vi "Read Joystick.vi"(8 "Joystick Deadbanded Value (default of 0.1)":dbl, 11 "Joystick L 1 DevRef":T1) -> (1 "Joystick L 2 X Axis":dbl, 2 "Joystick L 1 Y Axis":dbl, 3 "Joystick L 1 X Axis":dbl)   [LabVIEW 2014]
uses:
  <vilib>/Rock Robotics/WPI/Joystick/WPI_JoystickDevRef.ctl
  <vilib>/Rock Robotics/WPI/Joystick/WPI_JoystickDeviceEnum.ctl
  Global Variables.vi
  <vilib>/Rock Robotics/WPI/Joystick/WPI_JoystickGetSetRefNum.vi
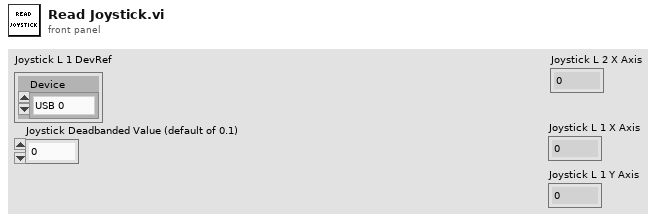
[diagram p1: front panel]
types:
  T1 = typedef "WPI_JoystickDevRef.ctl" = cluster{"Device":T2}
  T2 = typedef "WPI_JoystickDeviceEnum.ctl" = enum16{"USB 0", "USB 1", "USB 2", "USB 3", "USB 4", "USB 5"}
  T3 = cluster{"Buttons[0]":bool, "Buttons[1]":bool, "Buttons[2]":bool, "Buttons[3]":bool, "Buttons[4]":bool, "Buttons[5]":bool, "Buttons[6]":bool, "Buttons[7]":bool, "Buttons[8]":bool}
  T4 = cluster{"Axes[0]":dbl, "Axes[1]":dbl, "Axes[2]":dbl, "Axes[3]":dbl, "Axes[4]":dbl, "Axes[5]":dbl, "Axes[6]":dbl, "Axes[7]":dbl, "Axes[8]":dbl}
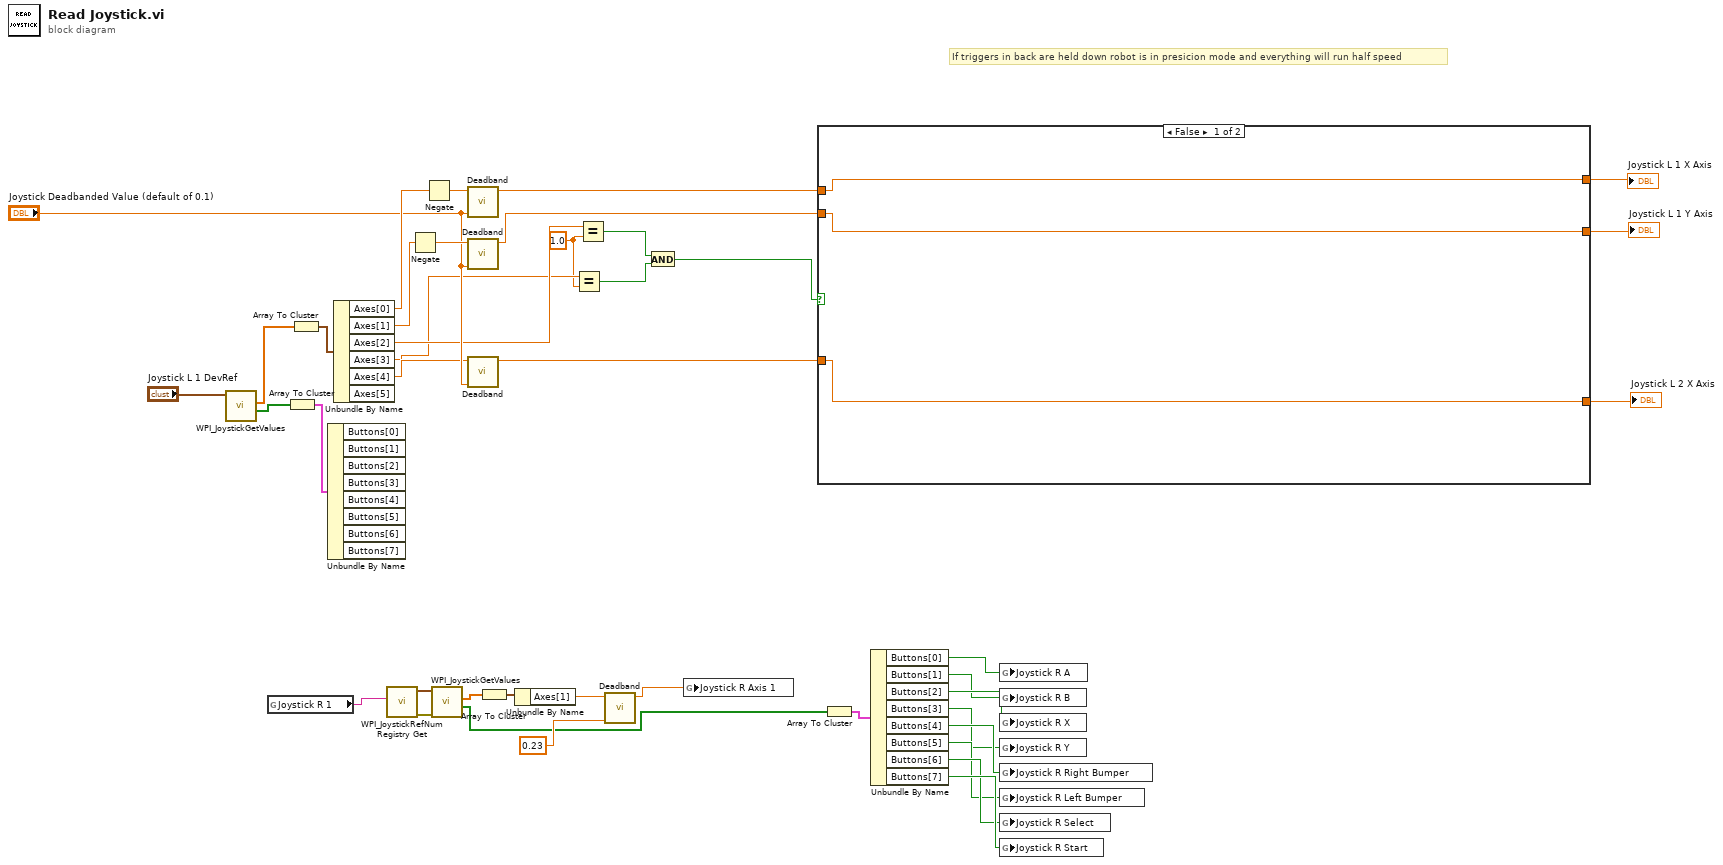
[diagram p0: block diagram]
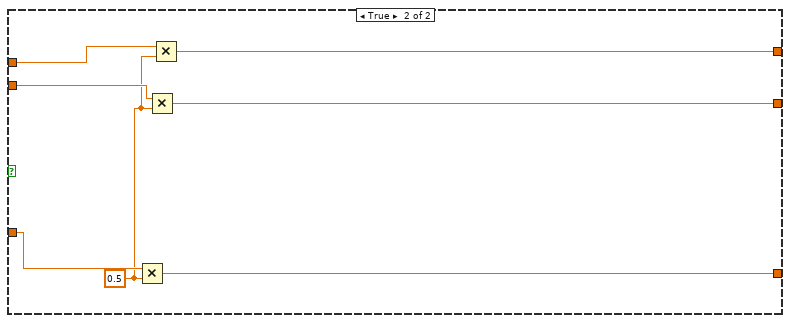
[diagram p2: hidden frame]
diagram:
  w10 = 1.0 ("y")
  # "If triggers in back are held down robot is in presicion mode and everything will run half speed"
  n1 = call <vilib>:"WPI_JoystickGetValues.vi"("JoystickDevRef"="Joystick L 1 DevRef") -> ("Buttons"=w38:bool[], "Axes"=w40:dbl[])  [unwired: 6 in, 3 out]
  n2 = global read "Global Variables.vi" "Joystick R 1"() -> (w29:string)
  n3 = Array To Cluster(array=w38) -> (cluster=w37:T3)
  n4 = Array To Cluster(array=w40) -> (cluster=w39:T4)
  n5 = Unbundle By Name(w37) -> ()  [unwired: 8 out]
  n6 = Unbundle By Name(w39) -> ("Axes[0]"=w36:dbl, "Axes[1]"=w33:dbl, "Axes[2]"=w12:dbl, "Axes[3]"=w11:dbl, "Axes[4]"=w13:dbl)  [unwired: 1 out]
  n7 = call <vilib>:"WPI_JoystickRefNum Registry Get.vi"("refnum name"=w29) -> ("error out"=w28:errorcluster, "JoystickDevRef"=w27:T1)  [unwired: 9 in]
  n8 = Negate(x=w33) -> (-x=w34:dbl)
  n9 = Negate(x=w36) -> (-x=w35:dbl)
  n10 = call <vilib>:"WPI_JoystickGetValues.vi"("error in (no error)"=w28, "JoystickDevRef"=w27) -> ("Buttons"=w15:bool[], "Axes"=w30:dbl[])  [unwired: 5 in, 3 out]
  n11 = call "Deadband.vi"("Value to Deadband (default of 0.1)"="Joystick Deadbanded Value (default of 0.1)", "Value"=w35) -> ("Deadbanded Value"=w4:dbl)  [unwired: 9 in]
  n12 = call "Deadband.vi"("Value to Deadband (default of 0.1)"="Joystick Deadbanded Value (default of 0.1)", "Value"=w34) -> ("Deadbanded Value"=w5:dbl)  [unwired: 9 in]
  n13 = call "Deadband.vi"("Value to Deadband (default of 0.1)"="Joystick Deadbanded Value (default of 0.1)", "Value"=w13) -> ("Deadbanded Value"=w6:dbl)  [unwired: 9 in]
  n14 = Array To Cluster(array=w30) -> (cluster=w31:T4)
  n15 = Unbundle By Name(w31) -> ("Axes[1]"=w25:dbl)
  n16 = Equal?(x=w11, y=w10) -> (x = y?=w8:bool)
  n17 = Equal?(x=w12, y=w10) -> (x = y?=w9:bool)
  n18 = call "Deadband.vi"("Value to Deadband (default of 0.1)"=0.23, "Value"=w25) -> ("Deadbanded Value"=w24:dbl)  [unwired: 9 in]
  n19 = And(x=w9, y=w8) -> (x .and. y?=w7:bool)
  n20 = global write "Global Variables.vi" "Joystick R Axis 1"(w24) -> ()
  n21 = case shown="False" w7 {
    tunnel: w6 -> [w42 w51]
    tunnel: w5 -> [w43 w50]
    tunnel: w4 -> [w44 w48]
    tunnel: [w44 w47] -> w3
    tunnel: [w43 w46] -> w2
    tunnel: [w42 w45] -> w1
    frame False {
    }
    frame True {
      w49 = 0.5 ("y")
      n22 = Multiply(x=w51, y=w49) -> (x*y=w45:dbl)
      n23 = Multiply(x=w50, y=w49) -> (x*y=w46:dbl)
      n24 = Multiply(x=w48, y=w49) -> (x*y=w47:dbl)
    }
  }
  "Joystick L 1 Y Axis" <- w2
  "Joystick L 1 X Axis" <- w3
  "Joystick L 2 X Axis" <- w1
  n25 = Array To Cluster(array=w15) -> (cluster=w16:T3)
  n26 = Unbundle By Name(w16) -> ("Buttons[0]"=w14:bool, "Buttons[1]"=w17:bool, "Buttons[2]"=w18:bool, "Buttons[3]"=w19:bool, "Buttons[4]"=w20:bool, "Buttons[5]"=w21:bool, "Buttons[6]"=w22:bool, "Buttons[7]"=w23:bool)
  n27 = global write "Global Variables.vi" "Joystick R A"(w14) -> ()
  n28 = global write "Global Variables.vi" "Joystick R B"(w17) -> ()
  n29 = global write "Global Variables.vi" "Joystick R X"(w18) -> ()
  n30 = global write "Global Variables.vi" "Joystick R Y"(w19) -> ()
  n31 = global write "Global Variables.vi" "Joystick R Right Bumper"(w20) -> ()
  n32 = global write "Global Variables.vi" "Joystick R Left Bumper"(w21) -> ()
  n33 = global write "Global Variables.vi" "Joystick R Select"(w22) -> ()
  n34 = global write "Global Variables.vi" "Joystick R Start"(w23) -> ()
